vi "Set Image.vi"(8 "error in (no error)":errorcluster, 10 "Picture":picture, 11 "Reference Control in":refnum<class "Reference Control.lvclass">) -> (0 "error out":errorcluster, 3 "Reference Control out":refnum<class "Reference Control.lvclass">)   [LabVIEW 2016, in "Reference Control.lvclass"]
uses:
  Reference Control.lvclass
  Reference Control.lvclass/Reference Control.ctl
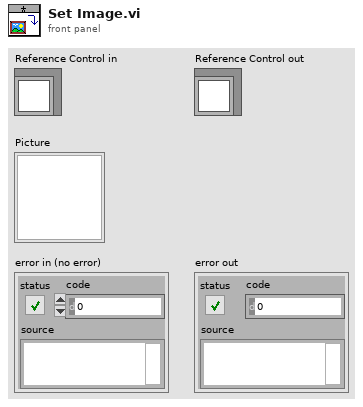
[diagram p1: front panel]
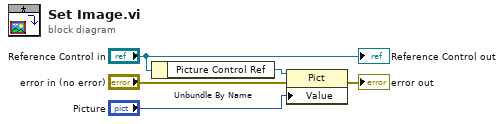
[diagram p0: block diagram]
diagram:
  n1 = Unbundle By Name("Reference Control in") -> ("Picture Control Ref"=w2:refnum<vi>)
  n2 = property on="Property Node" class="Pict"(reference=w2, error in="error in (no error)", "Value"="Picture") -> (error out=→"error out":errorcluster)  [unwired: 1 out]
  "Reference Control out" <- "Reference Control in"
